vi "FixedTrigger40Hz.vi"(8 "array in":bool[](array[boolean])=[FALSE, FALSE, FALSE, FALSE, FALSE, FALSE, FALSE, FALSE, FALSE, FALSE, FALSE, FALSE, FALSE], 9 "IO Module\\Synchronous Trigger Input":u8, 11 "Last? Input":bool) -> (0 "array out":bool[](array[boolean]), 1 "trigger out":bool[](array[boolean]))   [LabVIEW 2012]
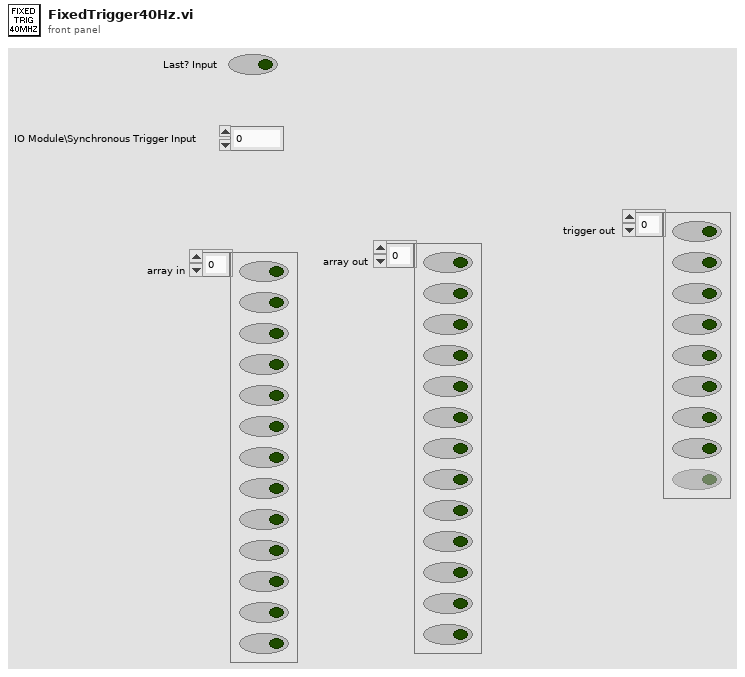
[diagram p1: front panel]
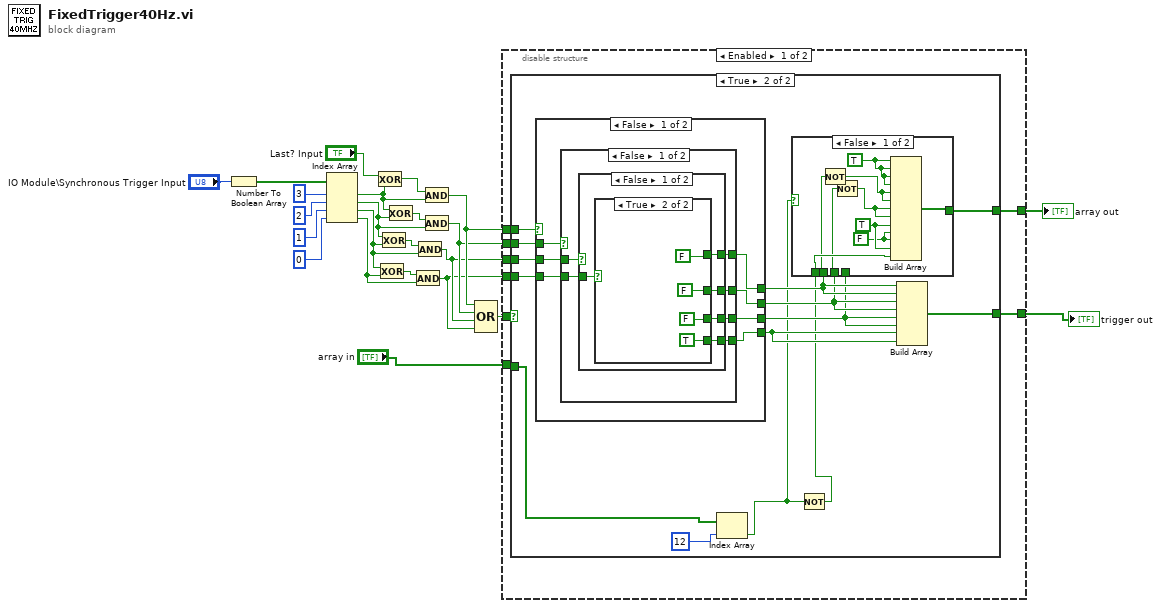
[diagram p0: block diagram]
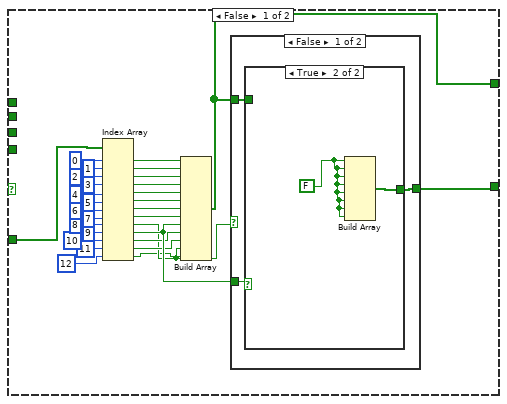
[diagram p2: hidden frame]
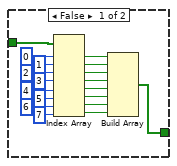
[diagram p3: hidden frame]
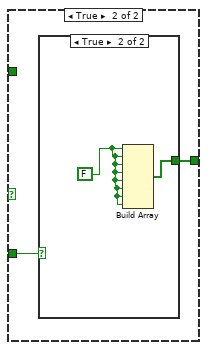
[diagram p4: hidden frame]
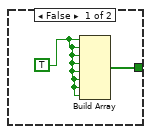
[diagram p5: hidden frame]
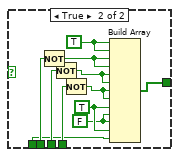
[diagram p6: hidden frame]
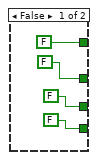
[diagram p7: hidden frame]
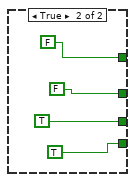
[diagram p8: hidden frame]
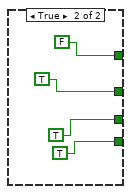
[diagram p9: hidden frame]
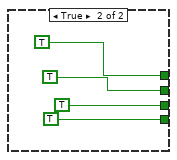
[diagram p10: hidden frame]
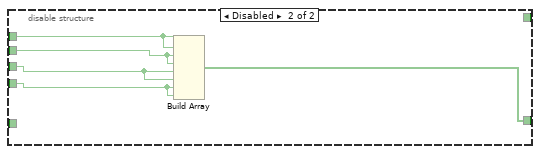
[diagram p11: hidden frame]
diagram:
  n1 = Number To Boolean Array(number="IO Module\\Synchronous Trigger Input") -> (Boolean array=w22:bool[])
  n2 = Index Array(array=w22, index #1=3, index #2=2, index #3=1, index #4=0) -> (element #1=w14:bool, element #2=w12:bool, element #3=w10:bool, element #4=w9:bool)
  n3 = Exclusive Or(1:w14, 2:"Last? Input") -> (0:w15:bool)
  n4 = Exclusive Or(1:w9, 2:w10) -> (0:w8:bool)
  n5 = Exclusive Or(1:w10, 2:w12) -> (0:w11:bool)
  n6 = Exclusive Or(1:w12, 2:w14) -> (0:w13:bool)
  n7 = And(x=w8, y=w9) -> (x .and. y?=w4:bool)
  n8 = And(x=w11, y=w10) -> (x .and. y?=w5:bool)
  n9 = And(x=w15, y=w14) -> (x .and. y?=w7:bool)
  n10 = And(x=w13, y=w12) -> (x .and. y?=w6:bool)
  n11 = Compound Arithmetic op=OR(w7, w6, w5, w4) -> (w3:bool)
  n12 = disable-structure shown="Enabled" {
    disable-tunnel: [w31 _] -> w20
    disable-tunnel: w7 -> [w30 w165]
    disable-tunnel: w6 -> [w29 w166]
    disable-tunnel: w5 -> [w28 w164]
    disable-tunnel: w4 -> [w27 w163]
    disable-tunnel: w3 -> [w26 _]
    disable-tunnel: "array in" -> [w25 _]
    disable-tunnel: [w24 w162] -> w1
    frame Enabled {
      n13 = case shown="True" w26 {
        tunnel: w30 -> [_ w103]
        tunnel: w29 -> [_ w102]
        tunnel: w28 -> [_ w101]
        tunnel: w27 -> [_ w95]
        tunnel: w25 -> [w45 w92]
        tunnel: [w35 w100] -> w24
        tunnel: [w34 w96] -> w31
        frame False {
          n14 = Index Array(array=w45, index #1=0 ("index"), index #2=1 ("index"), index #3=2 ("index"), index #4=3 ("index"), index #5=4 ("index"), index #6=5 ("index"), index #7=6 ("index"), index #8=7 ("index"), index #9=8 ("index"), index #10=9 ("index"), index #11=10 ("index"), index #12=11 ("index"), index #13=12 ("index")) -> (element #1=w40:bool, element #2=w52:bool, element #3=w51:bool, element #4=w50:bool, element #5=w49:bool, element #6=w48:bool, element #7=w47:bool, element #8=w46:bool, element #9=w36:bool, element #10=w39:bool, element #11=w38:bool, element #12=w37:bool, element #13=w33:bool)
          n15 = Build Array(w40, w52, w51, w50, w49, w48, w47, w46, w39, w38, w37, w36, w33) -> (w34:bool[])
          n16 = case shown="False" w36 {
            tunnel: w39 -> [w63 w85]
            tunnel: [w61 w84] -> w35
            tunnel: w34 -> [w62 _]
            frame False {
              n17 = case shown="True" w63 {
                tunnel: w62 -> [w65 _]
                tunnel: [w64 w82] -> w61
                frame False {
                  n18 = Index Array(array=w65, index #1=0 ("index"), index #2=1 ("index"), index #3=2 ("index"), index #4=3 ("index"), index #5=4 ("index"), index #6=5 ("index"), index #7=6 ("index"), index #8=7 ("index")) -> (element #1=w66:bool, element #2=w73:bool, element #3=w72:bool, element #4=w71:bool, element #5=w70:bool, element #6=w69:bool, element #7=w68:bool, element #8=w67:bool)
                  n19 = Build Array(w66, w73, w72, w71, w70, w69, w68, w67) -> (w64:bool[])
                }
                frame True {
                  w83 = FALSE
                  n20 = Build Array(w83, w83, w83, w83, w83, w83, w83, w83) -> (w82:bool[])
                }
              }
            }
            frame True {
              n21 = case shown="True" w85 {
                tunnel: [w86 w88] -> w84
                frame False {
                  w87 = TRUE
                  n22 = Build Array(w87, w87, w87, w87, w87, w87, w87, w87) -> (w86:bool[])
                }
                frame True {
                  w89 = FALSE
                  n23 = Build Array(w89, w89, w89, w89, w89, w89, w89, w89) -> (w88:bool[])
                }
              }
            }
          }
        }
        frame True {
          n24 = case shown="False" w103 {
            tunnel: w102 -> [w130 _]
            tunnel: w101 -> [w129 _]
            tunnel: w95 -> [w128 _]
            tunnel: [w125 TRUE] -> w99
            tunnel: [w126 TRUE] -> w98
            tunnel: [w127 TRUE] -> w97
            tunnel: [w124 TRUE] -> w94
            frame False {
              n25 = case shown="False" w130 {
                tunnel: w129 -> [w136 _]
                tunnel: w128 -> [w135 _]
                tunnel: [w134 TRUE] -> w124
                tunnel: [w133 TRUE] -> w127
                tunnel: [w132 TRUE] -> w126
                tunnel: [w131 FALSE] -> w125
                frame False {
                  n26 = case shown="False" w136 {
                    tunnel: w135 -> [w141 _]
                    tunnel: [w140 TRUE] -> w134
                    tunnel: [w139 TRUE] -> w133
                    tunnel: [w138 FALSE] -> w132
                    tunnel: [w137 FALSE] -> w131
                    frame False {
                      n27 = case shown="True" w141 {
                        tunnel: [FALSE TRUE] -> w140
                        tunnel: [FALSE FALSE] -> w139
                        tunnel: [FALSE FALSE] -> w138
                        tunnel: [FALSE FALSE] -> w137
                        frame False {
                        }
                        frame True {
                        }
                      }
                    }
                    frame True {
                    }
                  }
                }
                frame True {
                }
              }
            }
            frame True {
            }
          }
          n28 = Index Array(array=w92, index=12) -> (element=w90:bool)
          n29 = Not(x=w90) -> (.not. x?=w91:bool)
          n30 = case shown="False" w90 {
            tunnel: w99 -> [w109 w123]
            tunnel: w98 -> [w108 w122]
            tunnel: w97 -> [_ w121]
            tunnel: [w107 w120] -> w96
            tunnel: w91 -> [w110 w113]
            frame False {
              w111 = FALSE
              w112 = TRUE
              w106 = TRUE
              n31 = Not(x=w109) -> (.not. x?=w105:bool)
              n32 = Not(x=w108) -> (.not. x?=w104:bool)
              n33 = Build Array(w106, w106, w106, w106, w105, w105, w104, w104, w112, w111, w111, w112, w110) -> (w107:bool[])
            }
            frame True {
              w114 = FALSE
              w115 = TRUE
              w119 = TRUE
              n34 = Not(x=w123) -> (.not. x?=w118:bool)
              n35 = Not(x=w122) -> (.not. x?=w117:bool)
              n36 = Not(x=w121) -> (.not. x?=w116:bool)
              n37 = Build Array(w119, w119, w118, w118, w117, w117, w116, w116, w115, w114, w114, w115, w113) -> (w120:bool[])
            }
          }
          n38 = Build Array(w99, w99, w98, w98, w97, w97, w94, w94) -> (w100:bool[])
        }
      }
    }
    frame Disabled {
      n39 = Build Array(w165, w165, w166, w166, w164, w164, w163, w163) -> (w162:bool[])
    }
  }
  "array out" <- w20
  "trigger out" <- w1
